vi "Read LabVIEWHTTPClient_NET.vi"(8 "error in (no error)":errorcluster, 11 "REST Client_NET in":refnum<class "REST Client_NET.lvclass">) -> (0 "error out":errorcluster, 2 "LabVIEWHTTPClient_NET.lvlib:LabVIEWHTTPClient_NET":refnum<class "HttpClient_NET.lvclass">, 3 "REST Client_NET out":refnum<class "REST Client_NET.lvclass">)   [LabVIEW 2018, in "REST Client_NET.lvlib" / "REST Client_NET.lvclass"]
doc: "<b> </b> <b> </b>\nHttpClient_NET\nJustin Young - Viviota\nCopyright (c) 2021\nLicense: BSD"
uses:
  REST Client_NET.lvclass
  LabVIEWHTTPClient_NET/HttpClient_NET.lvclass
  REST Client_NET.lvclass/REST Client_NET.ctl
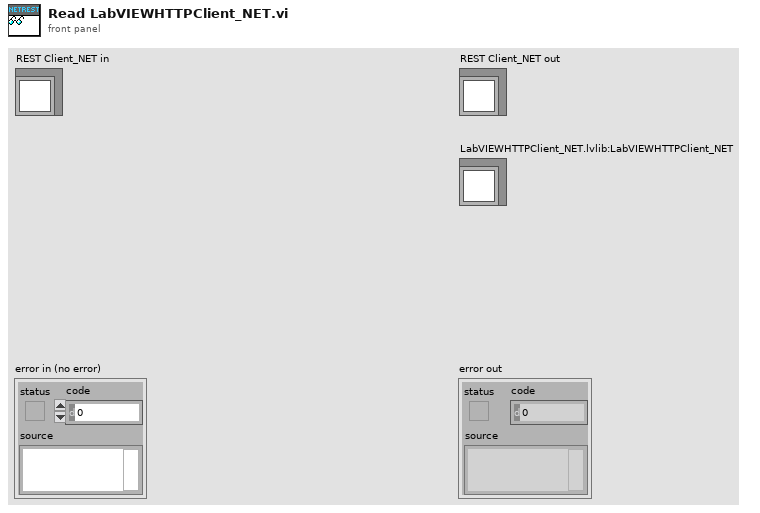
[diagram p1: front panel]
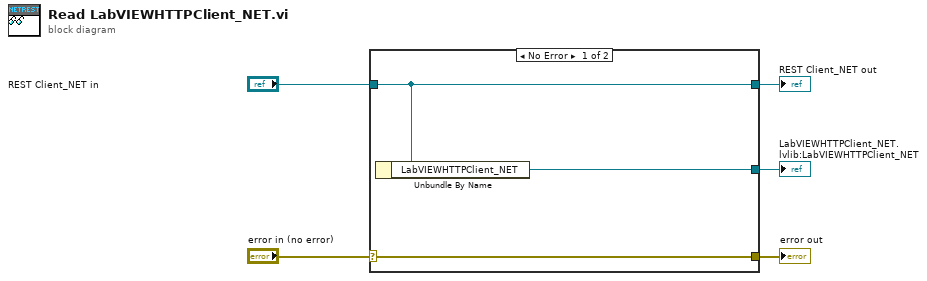
[diagram p0: block diagram]
diagram:
  n1 = case shown="No Error" "error in (no error)" {
    selector: "error in (no error)" -> [w8 w9]
    tunnel: [w8 w9] -> w4
    tunnel: [w7 w10] -> w2
    tunnel: "REST Client_NET in" -> [w7 w10]
    tunnel: [w6 _] -> w1
    frame No Error {
      n2 = Unbundle By Name(w7) -> ("LabVIEWHTTPClient_NET"=w6:refnum<class "HttpClient_NET.lvclass">)
    }
    frame Error {
    }
  }
  "error out" <- w4
  "REST Client_NET out" <- w2
  "LabVIEWHTTPClient_NET.lvlib:LabVIEWHTTPClient_NET" <- w1
